vi "Format Log XY Data.vi"(6 "Sweeping?":bool, 8 "error in (no error)":errorcluster, 9 "Y":waveform(dbl)[](array[waveform]), 10 "X":waveform(dbl)[](array[waveform]), 11 "Instrument.Lockin in":refnum<class "Instrument.Lockin.lvclass">) -> (0 "error out":errorcluster, 1 "Log Data":T1[](array[typedef]), 2 "Log Paths":string, 3 "Instrument.Lockin out":refnum<class "Instrument.Lockin.lvclass">, 4 "Times":timestamp[](array[timestamp]) format="%<%.6X\n%x>T")   [LabVIEW 2019, in "Instrument.Lockin.lvlib" / "Instrument.Lockin.lvclass"]
uses:
  Instrument.Lockin.lvclass
  Typedefs/Lockin.LogSweepXY--Cluster.ctl
  Instrument.Lockin.lvclass/Instrument.Lockin.ctl
  Instrument.DAQ/Instrument.DAQ.lvclass
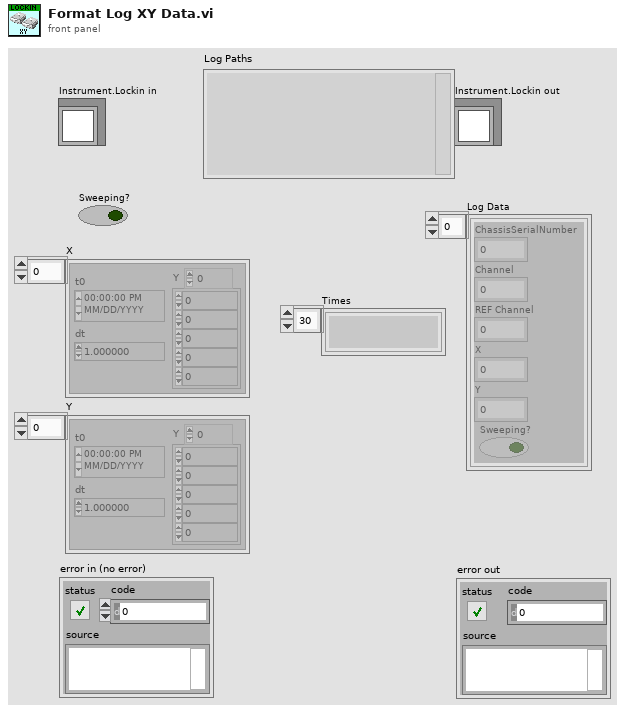
[diagram p1: front panel]
types:
  T1 = typedef "Instrument.Lockin.lvlib/Instrument.Lockin.lvclass/Lockin.LogSweepXY--Cluster.ctl" = cluster{"ChassisSerialNumber":u32, "Channel":i32, "REF Channel":i32, "X":dbl, "Y":dbl, "Sweeping?":bool}
  T2 = typedef "Instrument.Lockin.lvlib/Instrument.DAQ.lvclass/DeviceInfo--Cluster.ctl" = cluster{"DeviceName":string, "DevIsSimulated":bool, "DeviceSerialNumber":u32, "ProductType":string, "ProductCategory":i32, "ProductNumber":u32, "ChassisNumber":u32, "SlotNumber":u32, "ChassisName":string, "ChassisSerialNumber":u32}
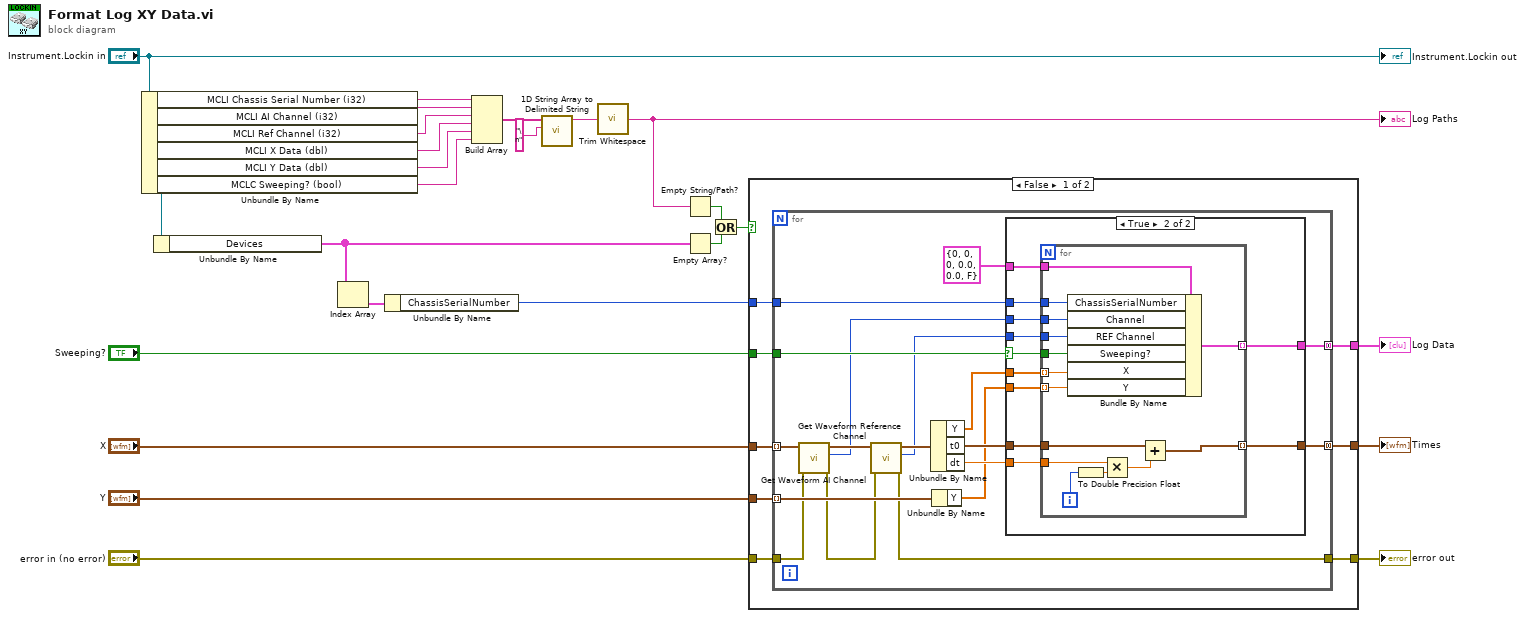
[diagram p0: block diagram]
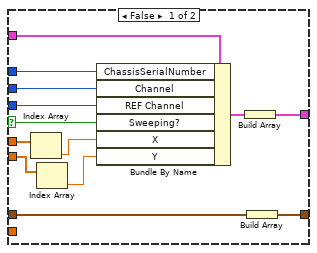
[diagram p2: hidden frame]
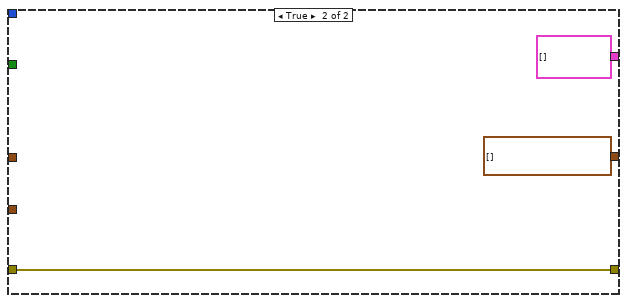
[diagram p3: hidden frame]
diagram:
  n1 = Unbundle By Name("Instrument.Lockin in") -> ("MCLI Chassis Serial Number (i32)"=w10:string, "MCLI AI Channel (i32)"=w15:string, "MCLI Ref Channel (i32)"=w14:string, "MCLI X Data (dbl)"=w13:string, "MCLI Y Data (dbl)"=w12:string, "MCLC Sweeping? (bool)"=w11:string)
  n2 = Unbundle By Name("Instrument.Lockin in") -> ("Devices"=w3:T2[])
  n3 = Index Array(array=w3) -> (element=w21:T2)  [unwired: 1 in]
  n4 = Unbundle By Name(w21) -> ("ChassisSerialNumber"=w20:u32)
  n5 = Build Array(w10, w15, w14, w13, w12, w11) -> (w9:string[])
  n6 = call <vilib>:"1D String Array to Delimited String.vi"("delimiter"="\n", "string array"=w9) -> ("delimited string"=w2:string)  [unwired: 9 in]
  n7 = call <vilib>:"Trim Whitespace.vi"("string"=w2) -> ("trimmed string"=w1:string)  [unwired: 1 in]
  "Log Paths" <- w1
  n8 = Empty String/Path?(string/path=w1) -> (empty?=w5:bool)
  n9 = Empty Array?(array=w3) -> (empty?=w6:bool)
  n10 = Or(x=w5, y=w6) -> (x .or. y?=w4:bool)
  n11 = case shown="False" w4 {
    tunnel: [w32 timestamp[] []] -> w24
    tunnel: "Sweeping?" -> [w31 _]
    tunnel: [w30 T1[] []] -> w22
    tunnel: w20 -> [w29 _]
    tunnel: "Y" -> [w28 _]
    tunnel: "X" -> [w27 _]
    tunnel: "error in (no error)" -> [w26 w90]
    tunnel: [w25 w90] -> w16
    frame False {
      n12 = for {
        tunnel: [w50] -> w32 mode=concatenating
        tunnel: w31 -> [w49]
        tunnel: [w48] -> w30 mode=concatenating
        tunnel: w29 -> [w47]
        tunnel: w28 -> [w46] mode=indexing
        tunnel: w27 -> [w39] mode=indexing
        tunnel: w26 -> [w36]
        tunnel: [w34] -> w25
        n13 = call "Get Waveform AI Channel.vi"("error in (no error)"=w36, "Reference in"=w39) -> ("error out"=w35:errorcluster, "AI Channel"=w37:i32, "Reference out"=w41:waveform(dbl))  [unwired: 7 in]
        n14 = call "Get Waveform Reference Channel.vi"("error in (no error)"=w35, "Reference in"=w41) -> ("error out"=w34:errorcluster, "Reference Channel"=w38:i32, "Reference out"=w40:waveform(dbl))  [unwired: 7 in]
        n15 = Unbundle By Name(w40) -> ("Y"=w42:dbl[], "t0"=w45:timestamp, "dt"=w44:dbl)
        n16 = Unbundle By Name(w46) -> ("Y"=w43:dbl[])
        n17 = case shown="True" w49 {
          selector: w49 -> [w57 w73]
          tunnel: [w56 w74] -> w50
          tunnel: w37 -> [w59 w72]
          tunnel: w44 -> [_ w71]
          tunnel: w45 -> [w55 w70]
          tunnel: [w62 w69] -> w48
          tunnel: w43 -> [w52 w68]
          tunnel: w38 -> [w58 w67]
          tunnel: T1 {"ChassisSerialNumber"=0, "Channel"=0, "REF Channel"=0, "X"=0.0, "Y"=0.0, "Sweeping?"=FALSE} ("cluster") -> [w63 w66]
          tunnel: w42 -> [w54 w65]
          tunnel: w47 -> [w60 w64]
          frame False {
            n18 = Index Array(array=w54) -> (element=w53:dbl)  [unwired: 1 in]
            n19 = Index Array(array=w52) -> (element=w51:dbl)  [unwired: 1 in]
            n20 = Bundle By Name(cluster=w63, "ChassisSerialNumber"=w60, "Channel"=w59, "REF Channel"=w58, "Sweeping?"=w57, "X"=w53, "Y"=w51) -> (w61:T1)
            n21 = Build Array(w61) -> (w62:T1[])
            n22 = Build Array(w55) -> (w56:timestamp[])
          }
          frame True {
            n23 = for {
              tunnel: w70 -> [w84]
              tunnel: w71 -> [w88]
              tunnel: [w75] -> w74 mode=indexing
              tunnel: w65 -> [w81] mode=indexing
              tunnel: w64 -> [w78]
              tunnel: w72 -> [w79]
              tunnel: w73 -> [w83]
              tunnel: [w82] -> w69 mode=indexing
              tunnel: w68 -> [w80] mode=indexing
              tunnel: w67 -> [w77]
              tunnel: w66 -> [w76]
              i -> [w87]
              n24 = Bundle By Name(cluster=w76, "ChassisSerialNumber"=w78, "Channel"=w79, "REF Channel"=w77, "Sweeping?"=w83, "X"=w81, "Y"=w80) -> (w82:T1)
              n25 = To Double Precision Float(number=w87) -> (double precision float=w86:dbl)
              n26 = Multiply(x=w88, y=w86) -> (x*y=w85:dbl)
              n27 = Add(x=w84, y=w85) -> (x+y=w75:timestamp)
            }
          }
        }
      }
    }
    frame True {
    }
  }
  "Times" <- w24
  "Log Data" <- w22
  "error out" <- w16
  "Instrument.Lockin out" <- "Instrument.Lockin in"
